vi "UpdateKeyboard.vi"(0 "View in":refnum<class "View.lvclass">, 1 "Letters":string[](array[string]), 2 "Result":u32[](array[colorbox]), 3 "error in (no error)":errorcluster) -> (7 "View out":refnum<class "View.lvclass">, 10 "error out":errorcluster)   [LabVIEW 2024, in "GUI.lvlib" / "View.lvclass"]
uses:
  View.lvclass
  View.lvclass/View.ctl
  TypeDefs/White.ctl
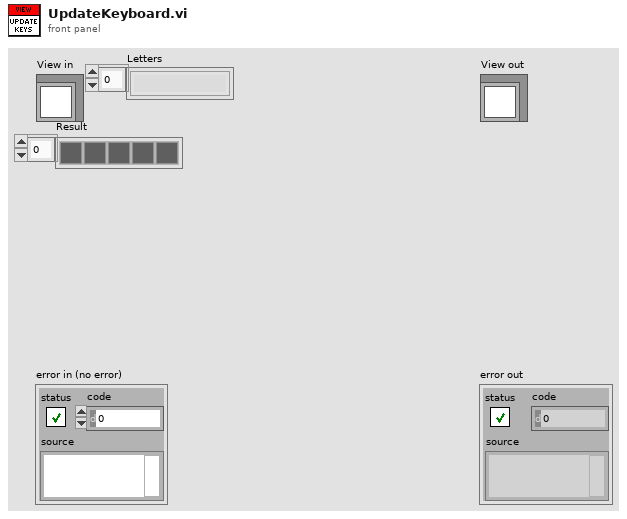
[diagram p1: front panel]
types:
  T1 = typedef "White.ctl" = u32
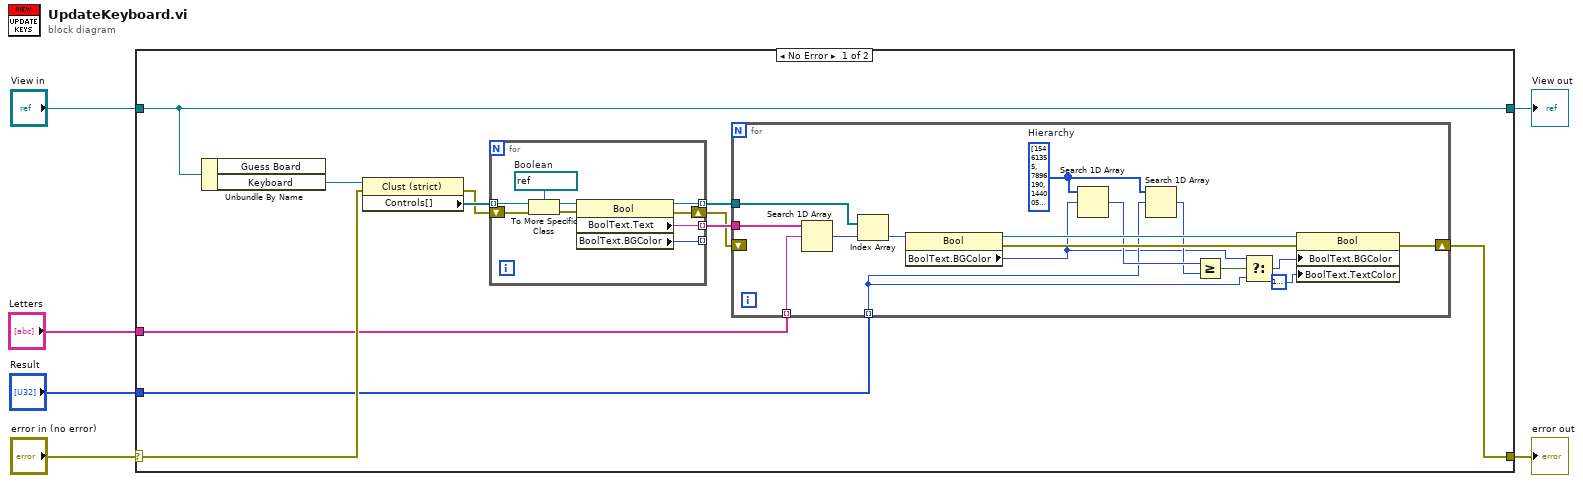
[diagram p0: block diagram]
diagram:
  n1 = case shown="No Error" "error in (no error)" {
    selector: "error in (no error)" -> [w13 w44]
    tunnel: [w7 w44] -> w5
    tunnel: [w17 w43] -> w3
    tunnel: "View in" -> [w17 w43]
    tunnel: "Result" -> [w9 _]
    tunnel: "Letters" -> [w12 _]
    frame No Error {
      n2 = Unbundle By Name(w17) -> ("Keyboard"=w16:refnum<vi>)  [unwired: 1 out]
      n3 = property class="Clust (strict)"(reference=w16, error in=w13) -> (error out=w14:errorcluster, "Controls[]"=w15:refnum<vi>[])  [unwired: 1 out]
      n4 = for {
        tunnel: w15 -> [w42] mode=indexing
        shift-right: [w38] -> w8
        shift-left: w14 -> [w37]
        tunnel: [w36] -> w11 mode=indexing
        tunnel: [w35] -> w10 mode=indexing
        tunnel: [w34] -> _ mode=indexing
        w41 = refnum<vi> refnum  # Boolean
        n5 = To More Specific Class(target class=w41, reference=w42, error in=w37) -> (specific class reference=w40:refnum<vi>, error out=w39:errorcluster)
        n6 = property class="Bool"(reference=w40, error in=w39) -> (reference out=w35:refnum<vi>, error out=w38:errorcluster, "BoolText.Text"=w36:string, "BoolText.BGColor"=w34:u32)
      }
      n7 = for {
        tunnel: w12 -> [w32] mode=indexing
        tunnel: w11 -> [w33]
        tunnel: w10 -> [w31]
        tunnel: w9 -> [w22] mode=indexing
        shift-right: [w19] -> w7
        shift-left: w8 -> [_]
        w26 = u32[] [15461355, 7896190, 14400581, 8173175]  # Hierarchy
        n8 = Search 1D Array(1D array=w33, element=w32) -> (index of element=w30:i32)  [unwired: 1 in]
        n9 = Index Array(array=w31, index=w30) -> (element=w29:refnum<vi>)
        n10 = property class="Bool"(reference=w29) -> (reference out=w28:refnum<vi>, error out=w27:errorcluster, "BoolText.BGColor"=w21:u32)  [unwired: 1 in]
        n11 = Search 1D Array(1D array=w26, element=w21) -> (index of element=w25:i32)  [unwired: 1 in]
        n12 = Search 1D Array(1D array=w26, element=w22) -> (index of element=w24:i32)  [unwired: 1 in]
        n13 = Greater Or Equal?(x=w25, y=w24) -> (x >= y?=w23:bool)
        n14 = Select(t=w21, s=w23, f=w22) -> (s? t:f=w20:u32)
        n15 = property class="Bool"(reference=w28, error in=w27, "BoolText.BGColor"=w20, "BoolText.TextColor"=T1 16777225 ("White")) -> (error out=w19:errorcluster)  [unwired: 1 out]
      }
    }
    frame Error {
    }
  }
  "error out" <- w5
  "View out" <- w3
